vi "Boiler Controller.vi"(8 "error in":errorcluster, 10 "Notifiers":T1, 11 "Message Queues":T2) -> (0 "error out":errorcluster)   [LabVIEW 2014]
uses:
  support/Message Queue/All Message Queues.ctl
  support/Message Queue/Message Cluster.ctl
  support/Notifiers/Notifiers.ctl
  controls/MHL UI Data.ctl
  controls/MHL Status.ctl
  support/Boiler System Globals.vi
  <vilib>/Utility/error.llb/Error Cluster From Error Code.vi
  <vilib>/ErrorRing/Error Ring.xnode
  support/Message Queue/Message Queue.lvlib
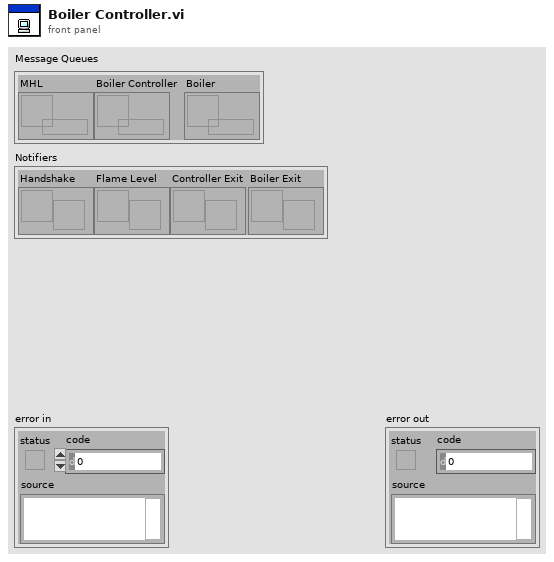
[diagram p1: front panel]
types:
  T1 = typedef "Notifiers.ctl" = cluster{"Handshake":refnum<notifier>, "Flame Level":refnum<notifier>, "Controller Exit":refnum<notifier>, "Boiler Exit":refnum<notifier>}
  T2 = typedef "Message Queue.lvlib/All Message Queues.ctl" = cluster{"MHL":refnum<queue>, "Boiler Controller":refnum<queue>, "Boiler":refnum<queue>}
  T3 = enum16{"open", "replace", "create", "open or create", "replace or create", "replace or create with confirmation"}
  T4 = typedef "MHL Status.ctl" = enum16{"Lockout", "Ready", "Pre-Purge", "Pre-Purge Complete", "Pilot On", "Boiler Running", "Shutdown", "Purge"}
  T5 = typedef "MHL UI Data.ctl" = cluster{"Status":string, "Fuel Control Valve":u32, "Primary Fan":bool, "Pilot Gas Valve":bool, "Pilot":bool, "Forced Draft Fan":bool, "MHL Status":T4}
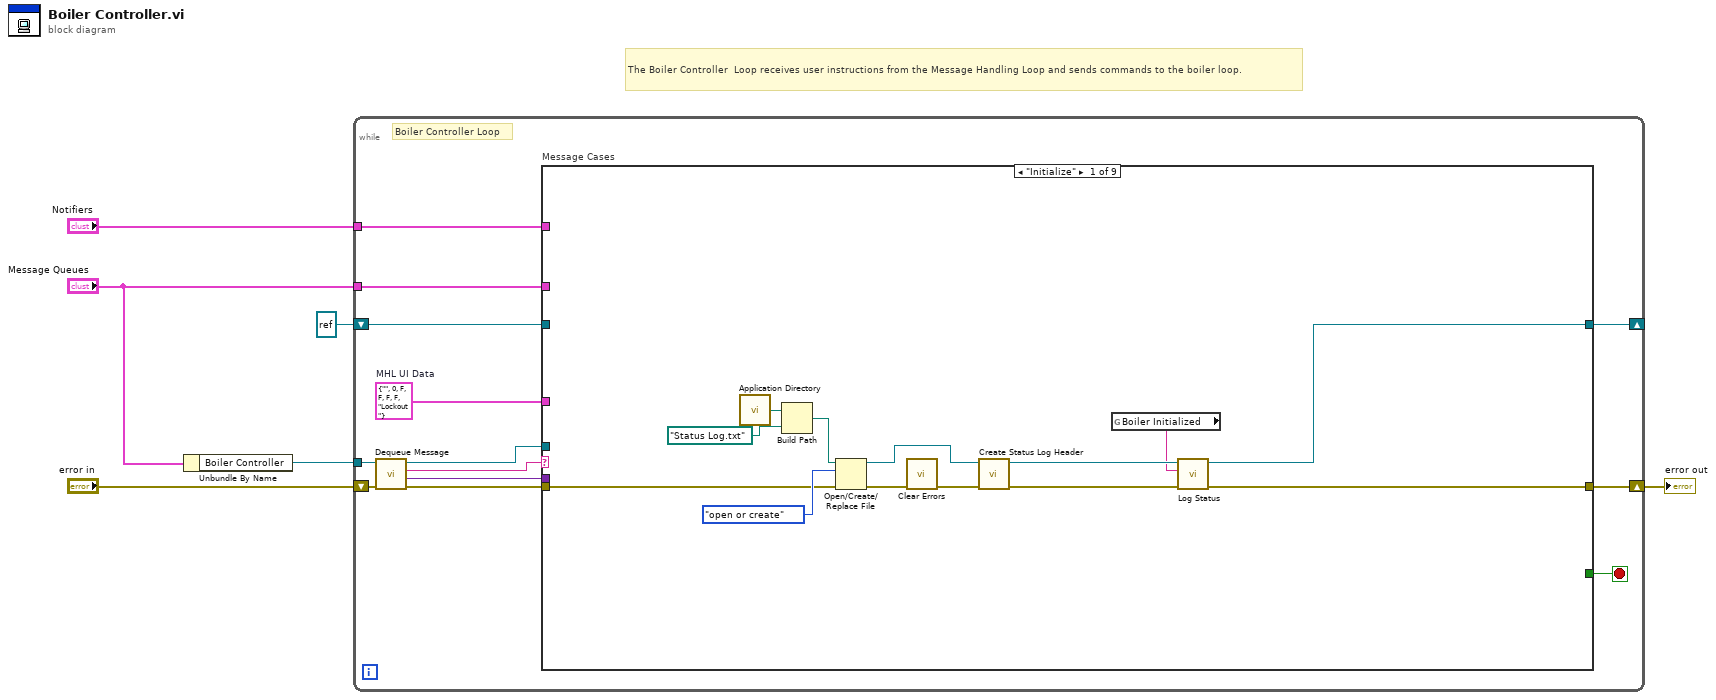
[diagram p0: block diagram]
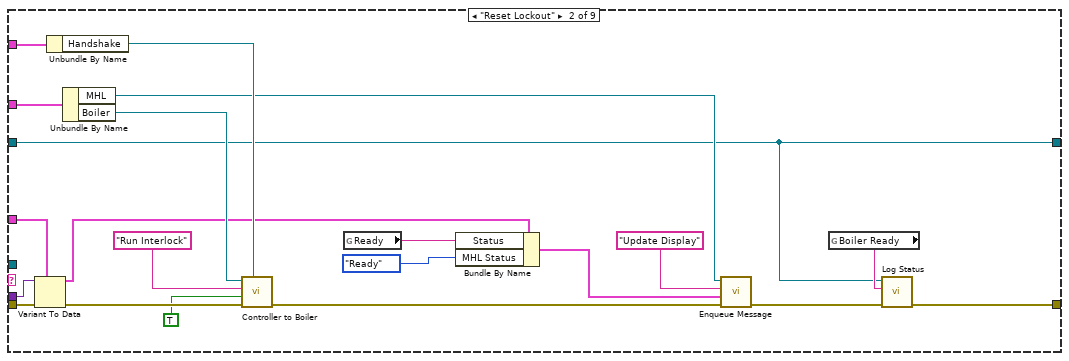
[diagram p2: hidden frame]
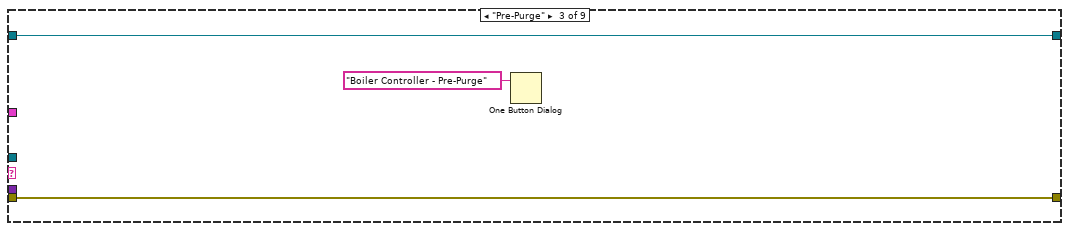
[diagram p3: hidden frame]
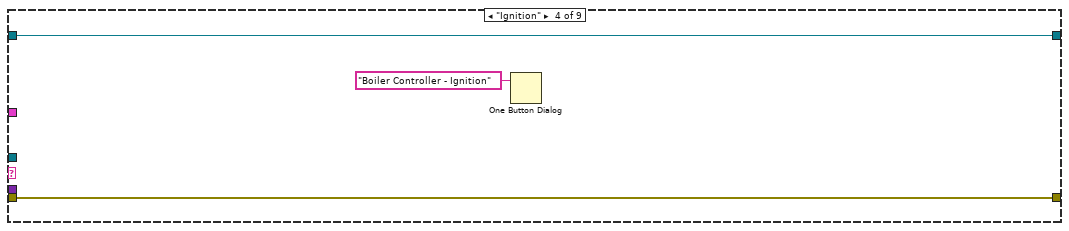
[diagram p4: hidden frame]
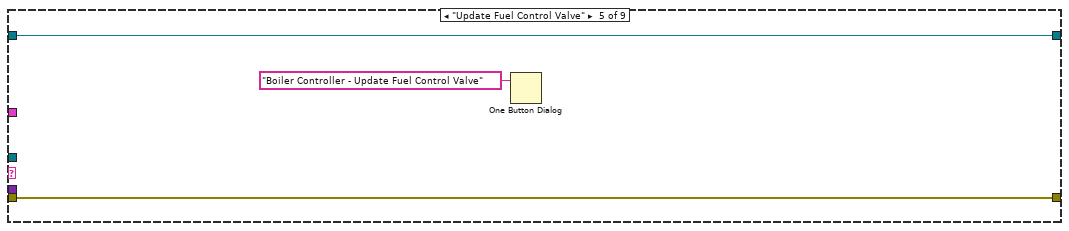
[diagram p5: hidden frame]
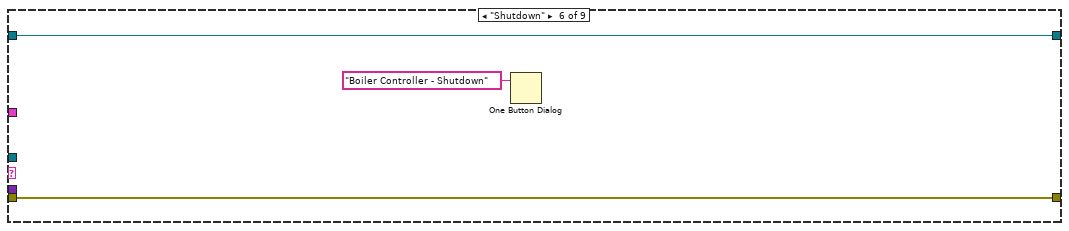
[diagram p6: hidden frame]
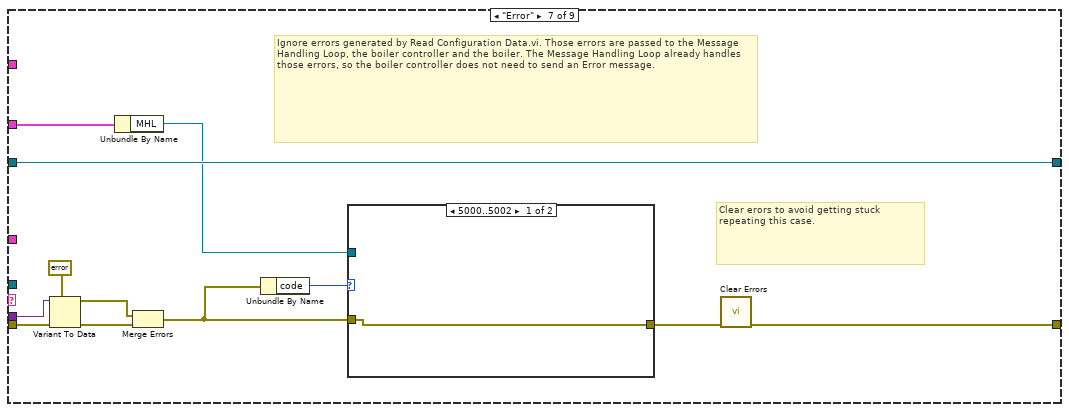
[diagram p7: hidden frame]
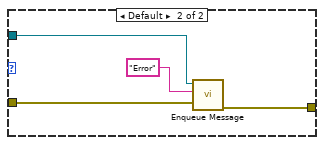
[diagram p8: hidden frame]
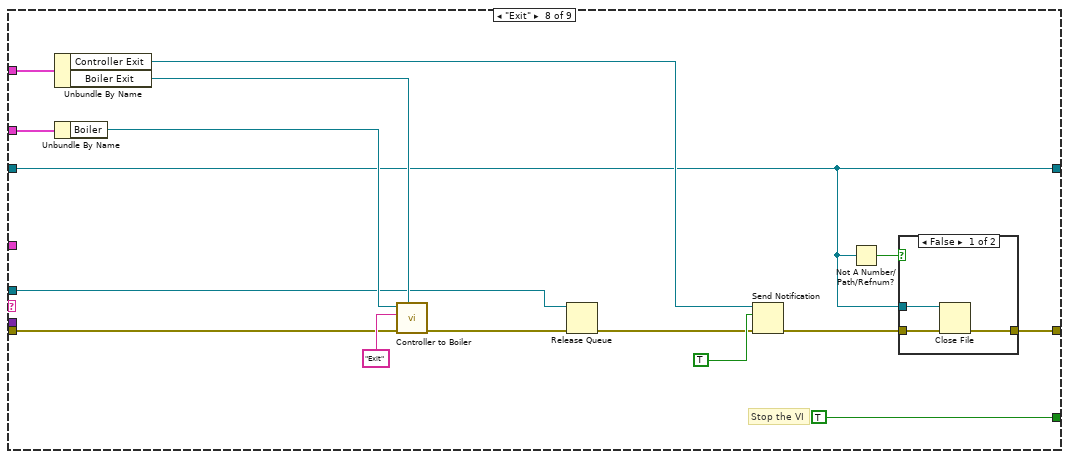
[diagram p9: hidden frame]
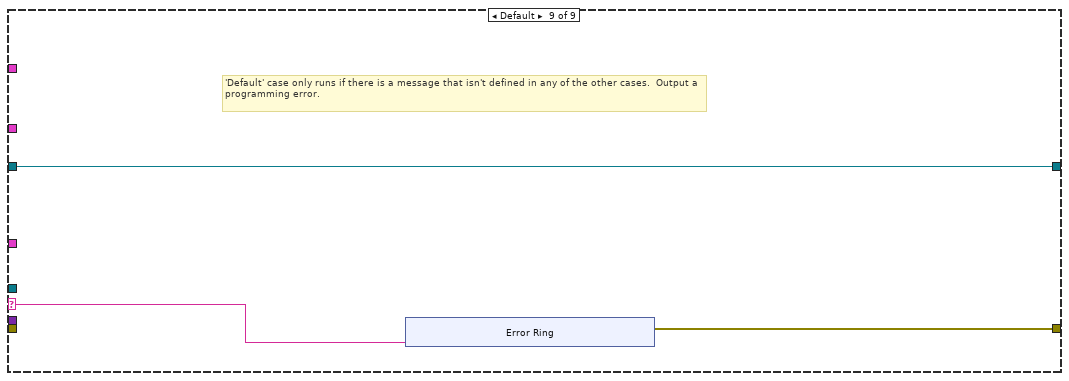
[diagram p11: hidden frame]
diagram:
  # "The Boiler Controller  Loop receives user instructions from the Message Handling Loop and sends commands to the boiler loop."
  n1 = Unbundle By Name("Message Queues") -> ("Boiler Controller"=w4:refnum<queue>)
  n2 = while {
    tunnel: w4 -> [w13]
    shift-right: [w12] -> w6
    shift-left: "error in" -> [w18]
    tunnel: "Message Queues" -> [w11]
    tunnel: "Notifiers" -> [w10]
    shift-right: [w9] -> _
    shift-left: refnum<file> refnum ("Log File Refnum Out") -> [w8]
    stop <- w19 stop-if-true
    w7 = T5 {"Status"="", "Fuel Control Valve"=0, "Primary Fan"=FALSE, "Pilot Gas Valve"=FALSE, "Pilot"=FALSE, "Forced Draft Fan"=FALSE, "MHL Status"=enum."Lockout"}  # MHL UI Data
    # "Boiler Controller Loop"
    n3 = call "Dequeue Message.vi"("error in (no error)"=w18, "Message Queue"=w13) -> ("error out"=w17:errorcluster, "Message Data"=w15:variant, "Message"=w16:string, "dup Message Queue"=w14:refnum<queue>)  [unwired: 6 in]
    n4 = case "Message Cases" shown="\"Initialize\"" w16 {
      selector: w16 -> [_ _ _ _ _ _ _ _ w104]
      tunnel: w14 -> [_ _ _ _ _ _ _ w91 _]
      tunnel: w17 -> [w22 w53 w56 w59 w62 w65 w76 w90 _]
      tunnel: [w23 w49 w56 w59 w62 w65 w68 w84 w105] -> w12
      tunnel: [_ _ _ _ _ _ _ TRUE _] -> w19
      tunnel: w15 -> [_ w48 _ _ _ _ w74 _ _]
      tunnel: w11 -> [_ w46 _ _ _ _ w77 w88 _]
      tunnel: w10 -> [_ w44 _ _ _ _ _ w87 _]
      tunnel: [w21 w34 w54 w57 w60 w63 w71 w83 w103] -> w9
      tunnel: w8 -> [_ w34 w54 w57 w60 w63 w71 w83 w103]
      tunnel: w7 -> [_ w47 _ _ _ _ _ _ _]
      frame "Initialize" {
        n5 = call <vilib>:"Application Directory.vi"() -> ("Application Directory"=w25:path)
        n6 = Build Path(base path=w25, name or relative path=path "Status Log.txt") -> (appended path=w29:path)
        n7 = Open/Create/Replace File(file path (use dialog)=w29, error in=w22, operation (0:open)=T3."open or create") -> (refnum out=w26:refnum<file>, error out=w27:errorcluster)  [unwired: 3 in, 1 out]
        n8 = call <vilib>:"Clear Errors.vi"("error in (no error)"=w27) -> ("error out"=w20:errorcluster)  [unwired: 5 in, 1 out]
        n9 = call "Create Status Log Header.vi"("error in"=w20, "Log File Refnum in"=w26) -> ("error out"=w32:errorcluster, "Log File Refnum out"=w31:refnum<file>)  [unwired: 8 in]
        n10 = global read "Boiler System Globals.vi" "Boiler Initialized"() -> (w30:string)
        n11 = call "Log Status.vi"("error in"=w32, "Event String"=w30, "Log File Refnum In"=w31) -> ("error out"=w23:errorcluster, "Log File Refnum Out"=w21:refnum<file>)  [unwired: 7 in]
      }
      frame "Reset Lockout" {
        n12 = Variant To Data(error in=w53, type=w47, Variant=w48) -> (data=w40:T5, error out=w52:errorcluster)
        n13 = Unbundle By Name(w44) -> ("Handshake"=w43:refnum<notifier>)
        n14 = Unbundle By Name(w46) -> ("MHL"=w36:refnum<queue>, "Boiler"=w45:refnum<queue>)
        n15 = call "Controller to Boiler.vi"("Notifier"=w43, "error in"=w52, "Message Data"=TRUE, "Message"="Run Interlock", "Boiler Queue in"=w45) -> ("error out"=w51:errorcluster)  [unwired: 4 in, 2 out]
        n16 = global read "Boiler System Globals.vi" "Ready"() -> (w39:string)
        n17 = Bundle By Name(cluster=w40, "Status"=w39, "MHL Status"=MHL_Status."Ready") -> (w38:T5)
        n18 = call "Enqueue Message.vi"("error in (no error)"=w51, "Message Data"=w38, "Message"="Update Display", "Message Queue"=w36) -> ("error out"=w50:errorcluster)  [unwired: 6 in, 1 out]
        n19 = global read "Boiler System Globals.vi" "Boiler Ready"() -> (w35:string)
        n20 = call "Log Status.vi"("error in"=w50, "Event String"=w35, "Log File Refnum In"=w34) -> ("error out"=w49:errorcluster)  [unwired: 7 in, 1 out]
      }
      frame "Pre-Purge" {
        n21 = One Button Dialog(message="Boiler Controller - Pre-Purge") -> ()  [unwired: 1 in, 1 out]
      }
      frame "Ignition" {
        n22 = One Button Dialog(message="Boiler Controller - Ignition") -> ()  [unwired: 1 in, 1 out]
      }
      frame "Update Fuel Control Valve" {
        n23 = One Button Dialog(message="Boiler Controller - Update Fuel Control Valve") -> ()  [unwired: 1 in, 1 out]
      }
      frame "Shutdown" {
        n24 = One Button Dialog(message="Boiler Controller - Shutdown") -> ()  [unwired: 1 in, 1 out]
      }
      frame "Error" {
        # "Ignore errors generated by Read Configuration Data.vi. Those errors are passed to the Message Handling Loop, the boiler controller and the boiler. The Message Handling Loop already handles those errors, so the boiler controller does not need to send an Error message."
        # "Clear erors to avoid getting stuck repeating this case."
        n25 = Variant To Data(error in=w76, type=errorcluster {"status"=FALSE, "code"=0, "source"=""} ("error out"), Variant=w74) -> (data=w72:errorcluster, error out=w73:errorcluster)
        n26 = Unbundle By Name(w77) -> ("MHL"=w67:refnum<queue>)
        n27 = Merge Errors(w72, w73) -> (w66:errorcluster)
        n28 = Unbundle By Name(w66) -> ("code"=w69:i32)
        n29 = case shown="5000..5002" w69 {
          tunnel: w67 -> [_ w81]
          tunnel: [w78 w80] -> w70
          tunnel: w66 -> [w78 w79]
          frame 5000..5002 {
          }
          frame Default {
            n30 = call "Enqueue Message.vi"("Message Data"=w79, "Message"="Error", "Message Queue"=w81) -> ("error out"=w80:errorcluster)  [unwired: 7 in, 1 out]
          }
        }
        n31 = call <vilib>:"Clear Errors.vi"("error in (no error)"=w70) -> ("error out"=w68:errorcluster)  [unwired: 5 in, 1 out]
      }
      frame "Exit" {
        # "Stop the VI"
        n32 = Unbundle By Name(w87) -> ("Controller Exit"=w93:refnum<notifier>, "Boiler Exit"=w95:refnum<notifier>)
        n33 = Unbundle By Name(w88) -> ("Boiler"=w92:refnum<queue>)
        n34 = call "Controller to Boiler.vi"("Notifier"=w95, "error in"=w90, "Message"="Exit", "Boiler Queue in"=w92) -> ("error out"=w98:errorcluster)  [unwired: 5 in, 2 out]
        n35 = Release Queue(queue=w91, error in (no error)=w98) -> (error out=w94:errorcluster)  [unwired: 1 in, 2 out]
        n36 = Send Notification(notification=TRUE, notifier=w93, error in (no error)=w94) -> (error out=w85:errorcluster)  [unwired: 1 out]
        n37 = Not A Number/Path/Refnum?(number/path/refnum=w83) -> (NaN/Path/Refnum?=w86:bool)
        n38 = case shown="False" w86 {
          tunnel: [w100 w102] -> w84
          tunnel: w85 -> [w101 w102]
          tunnel: w83 -> [w99 _]
          frame False {
            n39 = Close File(refnum=w99, error in=w101) -> (error out=w100:errorcluster)  [unwired: 1 out]
          }
          frame True {
          }
        }
      }
      frame Default {
        # "'Default' case only runs if there is a message that isn't defined in any of the other cases.  Output a programming error."
        n40 = xnode "Error Ring"("parameter 0"=w104) -> ("error out"=w105:errorcluster)
      }
    }
  }
  "error out" <- w6
